vi "Resample Blend.vi"(6 "Length":dbl=1.0, 8 "Speeds":T1={"maxV (fps)"=20.0, "Accel Limit (fps^2)"=20.0, "Initial V (fps)"=0.0, "Sample Period (s)"=0.02, "Jerk Limit (fps^3)"=0.0, "Jerk Distances"={"distance (ft)"=0.0, 0.0, 0.0}, "Jerk Distances"={"distance (ft)"=0.0, 0.0, 0.0}}, 9 "Initial Point":cluster{"x":dbl, "y":dbl, "th":dbl}={"x"=1.0, "y"=2.0, "th"=30.0}, 10 "Point Arrays":cluster{dbl[], dbl[], dbl[]}, 11 "Initial Acceleration":dbl format="%#_13g") -> (0 "Speeds Out":T1={"maxV (fps)"=20.0, "Accel Limit (fps^2)"=20.0, "Initial V (fps)"=0.0, "Sample Period (s)"=0.02, "Jerk Limit (fps^3)"=0.0, "Jerk Distances"={"distance (ft)"=0.0, 0.0, 0.0}, "Jerk Distances"={"distance (ft)"=0.0, 0.0, 0.0}}, 1 "Vel Points":cluster{dbl, dbl}[](array[cluster]), 2 "Points":cluster{dbl, dbl}[](array[cluster]), 3 "Indices":cluster{"Accel Index":i32, "Decel Index":i32}, 5 "Final Acceleration":dbl)   [LabVIEW 2020]
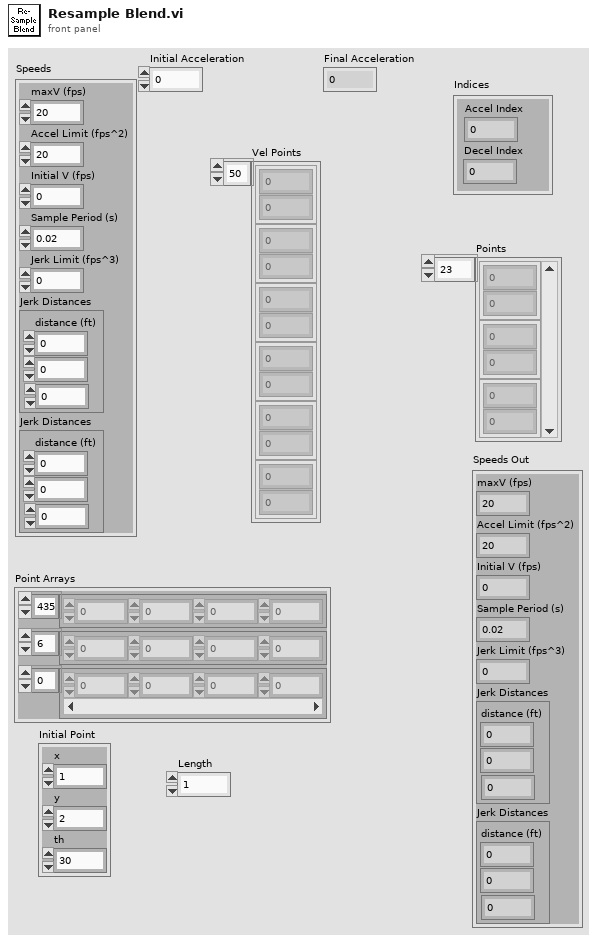
[diagram p1: front panel]
types:
  T1 = cluster{"maxV (fps)":dbl, "Accel Limit (fps^2)":dbl, "Initial V (fps)":dbl, "Sample Period (s)":dbl, "Jerk Limit (fps^3)":dbl, "Jerk Distances":cluster{"distance (ft)":dbl, dbl, dbl}, "Jerk Distances":cluster{"distance (ft)":dbl, dbl, dbl}}
  T2 = cluster{"Initial Acceleration":dbl, "Initial V (fps)":dbl}
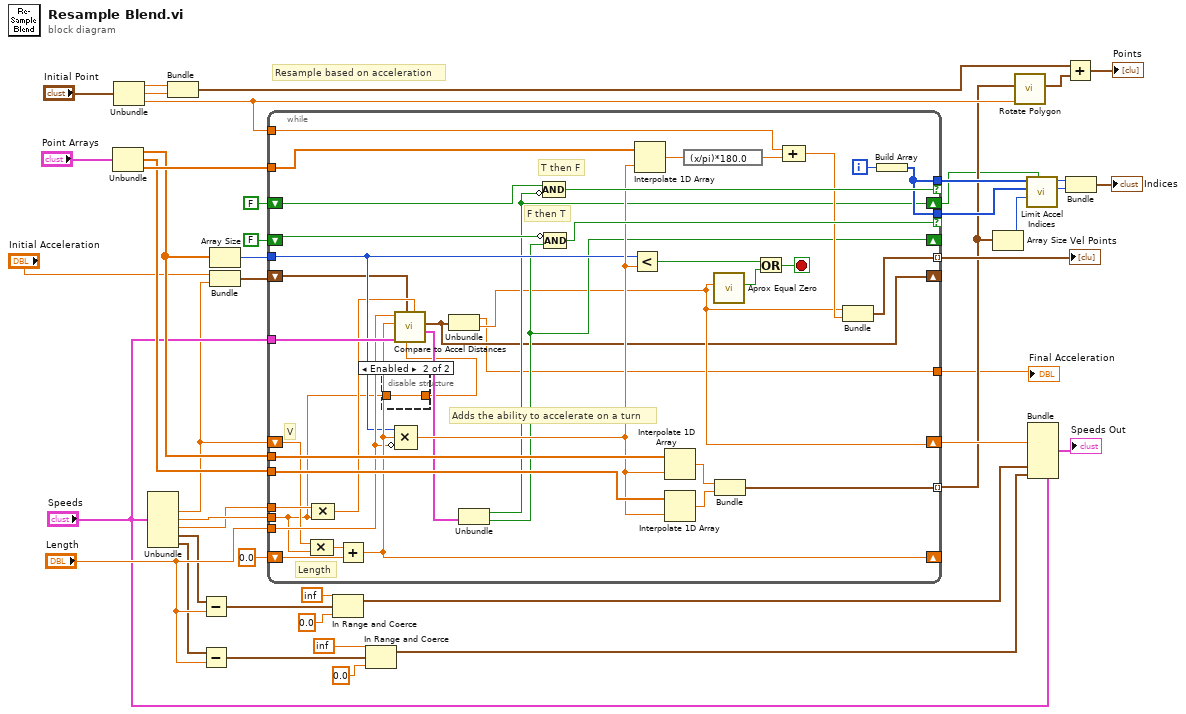
[diagram p0: block diagram]
diagram:
  # "Resample based on acceleration"
  n1 = Unbundle("Point Arrays") -> (w38:dbl[], w39:dbl[], w40:dbl[])
  n2 = Unbundle("Initial Point") -> ("x"=w35:dbl, "y"=w36:dbl, "th"=w34:dbl)
  n3 = Unbundle("Speeds") -> ("Initial V (fps)"=w3:dbl, "Sample Period (s)"=w44:dbl, "Jerk Limit (fps^3)"=w6:dbl, "Jerk Distances"=w10:cluster{"distance (ft)":dbl, dbl, dbl}, "Jerk Distances"=w11:cluster{"distance (ft)":dbl, dbl, dbl})  [unwired: 2 out]
  n4 = Bundle("x"=w35, "y"=w36) -> (w33:cluster{"x":dbl, "y":dbl})  [unwired: 1 in]
  n5 = Subtract(x=w10, y="Length") -> (x-y=w30:cluster{"distance (ft)":dbl, dbl, dbl})
  n6 = Subtract(x=w11, y="Length") -> (x-y=w26:cluster{"distance (ft)":dbl, dbl, dbl})
  n7 = Array Size(array=w38) -> (size(s)=w24:i32)
  n8 = Bundle("Initial Acceleration"="Initial Acceleration", "Initial V (fps)"=w3) -> (w5:T2)  [unwired: 1 in]
  n9 = while {
    tunnel: w38 -> [w83]
    tunnel: w39 -> [w82]
    tunnel: [w79] -> w17 mode=indexing
    tunnel: w44 -> [w46]
    shift-right: [w50] -> w43
    shift-left: w3 -> [w52]
    tunnel: w6 -> [w78]
    tunnel: w24 -> [w57]
    tunnel: w40 -> [w77]
    tunnel: w34 -> [w75]
    shift-right: [w54] -> w1
    shift-left: FALSE -> [w73]
    tunnel: [w61] -> w21 if=w72
    tunnel: "Length" -> [w59]
    tunnel: "Speeds" -> [w71]
    shift-right: [w53] -> _
    shift-left: FALSE -> [w70]
    tunnel: [w61] -> w20 if=w69
    tunnel: [w66] -> w22 mode=indexing
    shift-right: [w60] -> _
    shift-left: 0.0 -> [w64]
    shift-right: [w49] -> _
    shift-left: w5 -> [w48]
    tunnel: [w45] -> w2
    i -> [w62]
    stop <- w67 stop-if-true
    # "F then T"
    # "T then F"
    # "Adds the ability to accelerate on a turn"
    # "Length"
    # "V"
    n10 = Compound Arithmetic op=MULTIPLY(w52, w46) -> (w63:dbl)
    n11 = Compound Arithmetic op=MULTIPLY(w78, w46) -> (w51:dbl)
    n12 = Add(x=w63, y=w64) -> (x+y=w60:dbl)
    n13 = disable-structure shown="Enabled" {
      disable-tunnel: [_ w84] -> w47
      disable-tunnel: w46 -> [_ w84]
      frame Disabled {
      }
      frame Enabled {
      }
    }
    n14 = call "Compare to Accel Distances.vi"("dA"=w51, "Sample Period (s)"=w47, "Values"=w48, "Speeds"=w71, "Current  Length"=w60, "Total Segment Length"=w59) -> ("Ends"=w55:cluster{"Accel End":bool, "Decel End":bool}, "Values out"=w49:cluster{"accel":dbl, "velocity":dbl})  [unwired: 2 in, 2 out]
    n15 = Compound Arithmetic op=MULTIPLY(w57, w60, invert w59) -> (w58:dbl)
    n16 = Unbundle(w49) -> ("accel"=w45:dbl, "velocity"=w50:dbl)
    n17 = Unbundle(w55) -> ("Accel End"=w54:bool, "Decel End"=w53:bool)
    n18 = Compound Arithmetic op=AND(w73, invert w54) -> (w72:bool)
    n19 = Compound Arithmetic op=AND(invert w70, w53) -> (w69:bool)
    n20 = Less?(x=w57, y=w58) -> (x < y?=w68:bool)
    n21 = Interpolate 1D Array(1:w58, 2:w77) -> (0:w76:dbl)
    n22 = Interpolate 1D Array(1:w58, 2:w83) -> (0:w81:dbl)
    n23 = Interpolate 1D Array(1:w58, 2:w82) -> (0:w80:dbl)
    n24 = expression code="(x/pi)*180.0" ("radians to degrees")(w76) -> (w74:dbl)
    n25 = call "Aprox Equal Zero.vi"("maxV (fps)"=w50) -> ("Boolean"=w56:bool)  [unwired: 10 in]
    n26 = Bundle(w81, w80) -> (w79:cluster{dbl, dbl})  [unwired: 1 in]
    n27 = Or(x=w68, y=w56) -> (x .or. y?=w67:bool)
    n28 = Compound Arithmetic op=ADD(w75, w74) -> (w65:dbl)
    n29 = Bundle("velocity"=w50, w65) -> (w66:cluster{"velocity":dbl, dbl})  [unwired: 1 in]
    n30 = Build Array(w62) -> (w61:i32[])
  }
  "Vel Points" <- w22
  "Final Acceleration" <- w2
  n31 = In Range and Coerce(upper limit=inf, x=w30, lower limit=0.0) -> (coerced(x)=w8:cluster{"distance (ft)":dbl, dbl, dbl})  [unwired: 1 out]
  n32 = In Range and Coerce(upper limit=inf, x=w26, lower limit=0.0) -> (coerced(x)=w9:cluster{"distance (ft)":dbl, dbl, dbl})  [unwired: 1 out]
  n33 = Array Size(array=w17) -> (size(s)=w16:i32)
  n34 = call "Rotate Polygon.vi"("Angle"=w34, "polygon 2"=w17) -> ("polygon"=w32:cluster{dbl, dbl}[])  [unwired: 9 in]
  n35 = call "Limit Accel Indices.vi"("Last Accel"=w1, "Size"=w16, "Decel"=w20, "Accel"=w21) -> ("Decel Index"=w18:i32, "Accel Index"=w19:i32)  [unwired: 6 in]
  n36 = Bundle(cluster="Speeds", "Initial V (fps)"=w43, "Jerk Distances"=w8, "Jerk Distances"=w9) -> (→"Speeds Out":T1)  [unwired: 4 in]
  n37 = Add(x=w33, y=w32) -> (x+y=→"Points":cluster{dbl, dbl}[])
  n38 = Bundle("Accel Index"=w19, "Decel Index"=w18) -> (→"Indices":cluster{"Accel Index":i32, "Decel Index":i32})  [unwired: 1 in]
